vi "Validate Scalar Bitpacked Channel.vi"(8 "error in (no error)":errorcluster, 11 "Item Ref":T1 format="%.0x") -> (0 "error out":errorcluster, 2 "bitpacked":bool, 3 "item ref out":T1 format="%.0x")   [LabVIEW 2018, in "FPGA Addon System Explorer.lvlib"]
uses:
  FPGA Addon System Explorer.lvlib
  <vilib>/NI Veristand/Custom Device API/Custom Device Item Ref.ctl
  Addon Shared/SubVIs/Constants.vi
  <vilib>/NI Veristand/Custom Device API/Custom Device API.lvlib
  Addon Shared/FPGA Addon Shared.lvlib
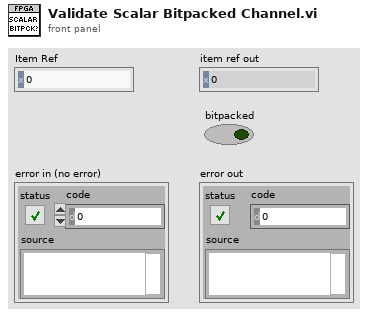
[diagram p1: front panel]
types:
  T1 = typedef "Custom Device API.lvlib/Custom Device Item Ref.ctl" = u64
  T2 = typedef "Custom Device API.lvlib/Custom Device Item Info.ctl" = cluster{"Name":string, "Is Channel":bool, "GUID":string, "Is Waveform":bool}
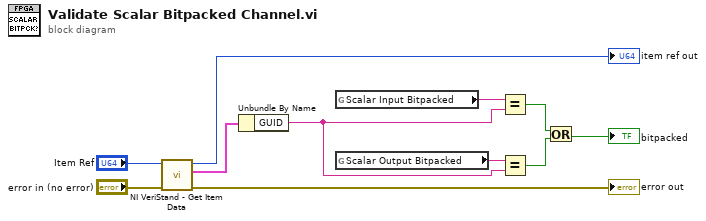
[diagram p0: block diagram]
diagram:
  n1 = call <vilib>:"NI VeriStand - Get Item Data.vi"("error in (no error)"="error in (no error)", "Item Ref in"="Item Ref") -> ("error out"=→"error out":errorcluster, "Item Info"=w5:T2, "Item Ref out"=→"item ref out":T1)  [unwired: 6 in, 1 out]
  n2 = Unbundle By Name(w5) -> ("GUID"=w8:string)
  n3 = global read "Constants.vi" "Scalar Input Bitpacked"() -> (w6:string)
  n4 = global read "Constants.vi" "Scalar Output Bitpacked"() -> (w7:string)
  n5 = Equal?(x=w6, y=w8) -> (x = y?=w9:bool)
  n6 = Equal?(x=w7, y=w8) -> (x = y?=w10:bool)
  n7 = Or(x=w9, y=w10) -> (x .or. y?=→"bitpacked":bool)
